vi "PopReportingRate.vi"(8 "ErrorArray In":errorcluster[](array[cluster]), 9 "Nominal Frequency (60)":u16(ring)=60 items=["50 Hz"=50, "60 Hz"=60]) -> (0 "ErrorArray Out":errorcluster[](array[cluster]))   [LabVIEW 2014, in "Framework.lvlib"]
uses:
  Framework.lvlib
  <userlib>/NIST/NISTErrorLib/NISTErrorLib.lvlib
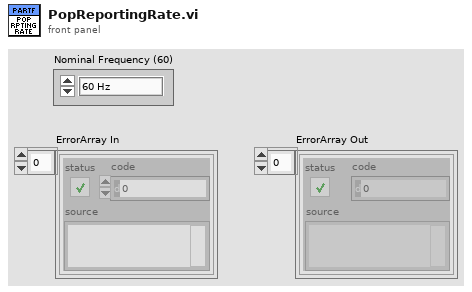
[diagram p1: front panel]
types:
  T1 = typedef "Framework.lvlib/clFrontPanelControlRefs.ctl" = cluster{"TestFilePathRef":refnum<vi>, "BusNumberRef":refnum<vi>, "NumberOfBusesRef":refnum<vi>, "EvtTypeRef":refnum<vi>, "EvtParamsRef":refnum<vi>, "EvtConfigRef":refnum<vi>, "StartTimeRef":refnum<vi>, "EndTimeRef":refnum<vi>, "PmuImpairTypeRef":refnum<vi>, "PmuImpairParamsRef":refnum<vi>, "NetImpairParamsRef":refnum<vi>, "FlagImpairTypeRef":refnum<vi>, "FlagImpairParamsRef":refnum<vi>, "NetImpairTypeRef":refnum<vi>, "OutputFileType":refnum<vi>, "PmuImpairConfigRef":refnum<vi>, "AppTypeRef":refnum<vi>, "ScriptPathRef":refnum<vi>, "ShowPanels?":refnum<vi>}
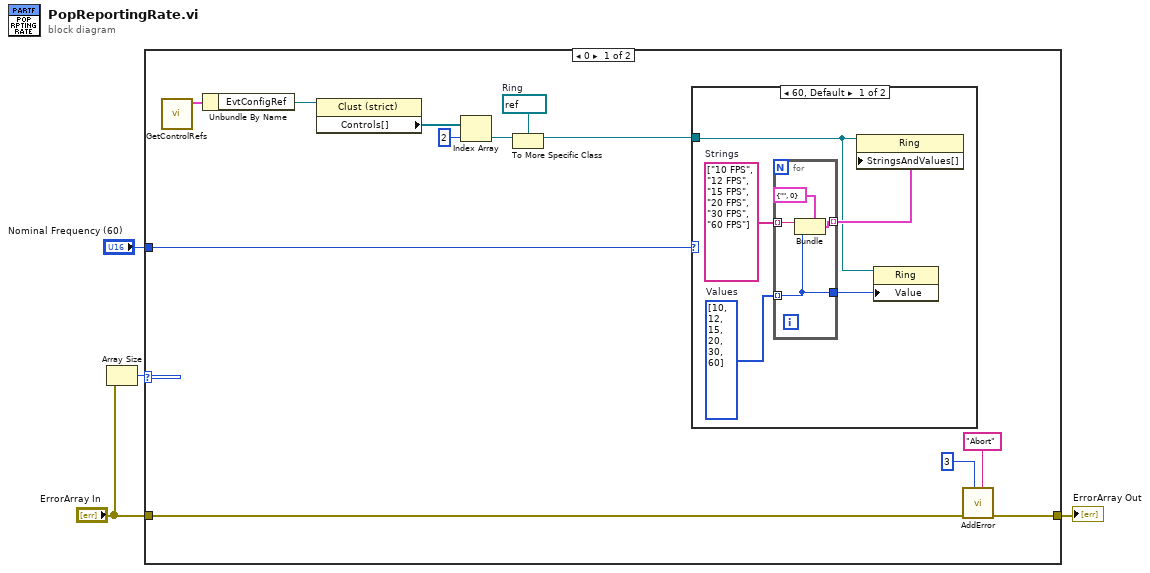
[diagram p0: block diagram]
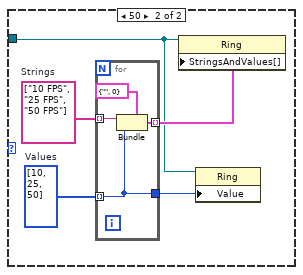
[diagram p2: hidden frame]
diagram:
  n1 = Array Size(array="ErrorArray In") -> (size(s)=w3:i32)
  n2 = case shown="0" w3 {
    tunnel: "ErrorArray In" -> [w14 w35]
    tunnel: [w13 w35] -> w4
    tunnel: "Nominal Frequency (60)" -> [w6 _]
    frame 0 {
      w7 = refnum<vi> refnum  # Ring
      n3 = call "GetControlRefs.vi"() -> ("clControlRefs Out"=w5:T1)  [unwired: 11 in]
      n4 = Unbundle By Name(w5) -> ("EvtConfigRef"=w12:refnum<vi>)
      n5 = property class="Clust (strict)"(reference=w12) -> ("Controls[]"=w9:refnum<vi>[])  [unwired: 1 in, 2 out]
      n6 = Index Array(array=w9, index=2) -> (element=w10:refnum<vi>)
      n7 = To More Specific Class(target class=w7, reference=w10) -> (specific class reference=w8:refnum<vi>)  [unwired: 1 in, 1 out]
      n8 = case shown="60, Default" w6 {
        tunnel: w8 -> [w19 w27]
        frame 60, Default {
          w17 = u16[] [10, 12, 15, 20, 30, 60]  # Values
          w18 = string[] ["10 FPS", "12 FPS", "15 FPS", "20 FPS", "30 FPS", "60 FPS"]  # Strings
          n9 = for {
            tunnel: w18 -> [w25] mode=indexing
            tunnel: w17 -> [w22] mode=indexing
            tunnel: [w24] -> w21 mode=indexing
            tunnel: [w22] -> w20
            n10 = Bundle(cluster=cluster{string, u16} {"", 0}, w25, w22) -> (w24:cluster{string, u16})
          }
          n11 = property class="Ring"(reference=w19, "StringsAndValues[]"=w21) -> ()  [unwired: 1 in, 2 out]
          n12 = property class="Ring"(reference=w19, "Value"=w20) -> ()  [unwired: 1 in, 2 out]
        }
        frame 50 {
          w29 = u16[] [10, 25, 50]  # Values
          w30 = string[] ["10 FPS", "25 FPS", "50 FPS"]  # Strings
          n13 = for {
            tunnel: w30 -> [w34] mode=indexing
            tunnel: w29 -> [w31] mode=indexing
            tunnel: [w33] -> w28 mode=indexing
            tunnel: [w31] -> w26
            n14 = Bundle(cluster=cluster{string, u16} {"", 0}, w34, w31) -> (w33:cluster{string, u16})
          }
          n15 = property class="Ring"(reference=w27, "StringsAndValues[]"=w28) -> ()  [unwired: 1 in, 2 out]
          n16 = property class="Ring"(reference=w27, "Value"=w26) -> ()  [unwired: 1 in, 2 out]
        }
      }
      n17 = call <userlib>:"AddError.vi"("Severity"="Abort" ("String"), "Priority"=u8 3, "ErrorArray"=w14) -> ("ErrorArray"=w13:errorcluster[])  [unwired: 7 in, 1 out]
    }
    frame 1, Default {
    }
  }
  "ErrorArray Out" <- w4
